vi "HFRR ADV v013 new software.vi"() -> ()   [LabVIEW 2025] (continued)
              n1464 = local write "FRIC. FORCE :"(w1751) -> ()
            }
            frame 1 {
              n1465 = local write "TEMPERATURE :"(w1752) -> ()
            }
            frame 2 {
              n1466 = local write "HUMIDITY:"(w1753) -> ()
            }
            frame 3 {
              n1467 = local write "AIR TEMPERATURE :"(w1754) -> ()
            }
            frame 4 {
              n1468 = local write "Com Port 1"(w1755) -> ()
            }
            frame 5 {
              n1469 = local write "Com Port 2"(w1756) -> ()
              n1470 = local write "visa due"(w1756) -> ()
            }
            frame 6 {
              n1471 = String To Path(string=w1757) -> (path=w1758:path)
              n1472 = local write "File Path"(w1758) -> ()
              "String" <- w1757
            }
            frame 7 {
              n1473 = local write "DISPLACEMENT :"(w1759) -> ()
            }
            frame 8 {
              n1474 = local write "STROKE GAIN :"(w1760) -> ()
            }
            frame 9 {
            }
            frame 10 {
              n1475 = local write "Language Selection"(w1761) -> ()
            }
            frame 11 {
              n1476 = local write "CH-POWER +"(w1762) -> ()
            }
            frame 12 {
              n1477 = local write "CH-POWER -"(w1763) -> ()
            }
            frame 13 {
              n1478 = local write "CH-HEATER"(w1764) -> ()
            }
            frame 14 {
              n1479 = local write "CH-HUMIDITY WET"(w1765) -> ()
            }
            frame 15 {
              n1480 = local write "CH-HUMIDITY DRY"(w1766) -> ()
            }
            frame 16 {
            }
            frame 17 {
              n1481 = local write "AIR TEMP INTERCEPT:"(w1767) -> ()
            }
            frame 18 {
              n1482 = local write "TEMP INTERCEPT:"(w1768) -> ()
            }
            frame 21 {
              n1483 = local write "S.NO"(w1769) -> ()
            }
            frame 22 {
              n1484 = local write "Com Port 3"(w1770) -> ()
            }
            frame 20 {
              n1485 = local write "Camera Port :"(w1771) -> ()
            }
            frame 19 {
              n1486 = local write "C3 :"(w1772) -> ()
            }
            frame 23, Default {
            }
          }
        }
      }
    }
    n1487 = Select(t=u32 2500 ("milliseconds to wait"), s=w1725, f=u32 500 ("milliseconds to wait")) -> (s? t:f=w1723:u32)
    n1488 = Multiply(x=w1728, y=w1723) -> (x*y=w1730:dbl)
    n1489 = property on="Time slide" class="Slide (strict)"("Visible"=w1719) -> ()  [unwired: 2 in, 2 out]
    n1490 = call "Elapsed Time2"("Time Target (s)"=w1730, "Auto Reset"=TRUE) -> ("Time has Elapsed"=w1720:bool)  [unwired: 10 in, 7 out]
    n1491 = case shown="True" w1720 {
      frame False {
      }
      frame True {
        n1492 = stacked-sequence {
          frame #0 {
            # "DATA PROCESSING"
            # "115 mV/N"
            n1493 = local read "Sample Temperature"() -> (w1775:dbl)
            n1494 = local read "RH Numeric:"() -> (w1782:dbl)
            n1495 = local read "HUMIDITY:"() -> (w1783:dbl)
            n1496 = local read "FRICVALZ"() -> (w1794:dbl)
            n1497 = local read "Friction"() -> (w1778:dbl)
            n1498 = Multiply(x=w1782, y=w1783) -> (x*y=→"Humidity ( %RH )" →"Hum" →"Hum 2":dbl)
            n1499 = call <vilib>:"Mean PtByPt.vi"("x"=w1775, "sample length"=100) -> ("mean"=w1774:dbl)  [unwired: 2 in, 1 out]
            "TEMP 2" <- w1774
            "TEMP 3" <- w1774
            n1500 = Subtract(x=w1778, y=w1794) -> (x-y=w1789:dbl)
            "FF 2" <- w1789
            "FF 4" <- w1789
            n1501 = local read "Ambient Temperature"() -> (→"AIR TEMP":dbl)
            n1502 = local read "TEMP"() -> (w1793:dbl)
            n1503 = local write "FF 3"(w1789) -> ()
            n1504 = Compound Arithmetic op=OR("FRICVALZ 4", "FRICVALZ 3", "FRICVALZ 2") -> (w1785:bool)
            n1505 = case shown="True" w1785 {
              tunnel: w1778 -> [_ w1800]
              frame False {
              }
              frame True {
                w1799 = FALSE ("FRICVALZ")
                n1506 = local write "FRICVALZ 3"(w1799) -> ()
                n1507 = local write "FRICVALZ 2"(w1799) -> ()
                n1508 = local write "FRICVALZ 4"(w1799) -> ()
                "FRICVALZ" <- w1800
              }
            }
            n1509 = Not A Number/Path/Refnum?(number/path/refnum=w1793) -> (NaN/Path/Refnum?=w1792:bool)
            n1510 = Not A Number/Path/Refnum?(number/path/refnum=w1789) -> (NaN/Path/Refnum?=w1791:bool)
            n1511 = Divide(x=w1789, y=1.96) -> (x/y=w1786:dbl)
            n1512 = Compound Arithmetic op=OR(w1792, w1791) -> (w1790:bool)
            n1513 = Not A Number/Path/Refnum?(number/path/refnum=w1786) -> (NaN/Path/Refnum?=w1787:bool)
            n1514 = case shown="True" w1790 {
              frame False {
              }
              frame True {
                n1515 = local write "TEMP"(0.0 ("TEMP")) -> ()
                n1516 = local write "FF 2"(0.0 ("FF 2")) -> ()
                n1517 = local write "reinit"(TRUE ("reinit")) -> ()
              }
            }
            n1518 = local write "TEMP"(w1774) -> ()
            n1519 = Select(t=0.0, s=w1787, f=w1786) -> (s? t:f=w1777:dbl)
            "COF 2" <- w1777
            n1520 = local write "COF 3"(w1777) -> ()
          }
        }
      }
    }
    n1521 = Wait (ms)(milliseconds to wait=u32 50) -> ()  [unwired: 1 out]
    n1522 = local read "Quit"() -> (w1712:bool)
    "Rate" <- 2500.0 ("No of Samples")
  }
  n1523 = while {
    tunnel: w57 -> [_]
    tunnel: [w1827] -> _
    tunnel: [w1803] -> w56
    i -> [w1827]
    stop <- w1803 stop-if-true
    # "C:\\LAB-IQ-NXT\\Scar View.exe"
    n1524 = local read "OK Button 16"() -> (w1816:bool)
    n1525 = local read "Main Tab"() -> (w1809:T2)
    n1526 = local read "service 3"() -> (w1810:bool)
    n1527 = local read "OPEN 6"() -> (w1812:bool)
    n1528 = local read "EDIT 2"() -> (w1814:bool)
    n1529 = flat-sequence {
      frame #0 {
        n1530 = local read "SAVE 2"() -> (w2429:bool)
        n1531 = stacked-sequence {
          frame #0 {
            n1532 = local read "EDIT"() -> (w2483:bool)
            n1533 = case shown="True" w2483 {
              tunnel: [u8 2 ("Disabled") u8 0 ("Disabled")] -> _
              frame False {
                w2485 = FALSE
                n1534 = local write "Password"("") -> ()
                n1535 = property on="SrvM CP" class="Bool (strict)"("Visible"=w2485) -> ()  [unwired: 2 in, 2 out]
                n1536 = property on="message" class="Str"("Visible"=w2485) -> ()  [unwired: 2 in, 2 out]
                n1537 = local write "x = y?"(w2485) -> ()
                n1538 = property on="Password" class="Str"("Visible"=w2485) -> ()  [unwired: 2 in, 2 out]
                n1539 = property on="ENTER THE NEW PASSWORD" class="Str"("Visible"=w2485) -> ()  [unwired: 2 in, 2 out]
                n1540 = property on="ENTER CURRENT PASSWORD" class="Str"("Visible"=w2485) -> ()  [unwired: 2 in, 2 out]
                n1541 = local write "SrvM CP"(w2485) -> ()
              }
              frame True {
                w2488 = TRUE
                n1542 = property on="SrvM CP" class="Bool (strict)"("Visible"=w2488) -> ()  [unwired: 2 in, 2 out]
                n1543 = property on="Password" class="Str"("Visible"=w2488) -> ()  [unwired: 2 in, 2 out]
              }
            }
            "dipl pwd" <- "@143$\n" ("dipl pwd")
          }
          frame #1 {
            # "Gain password"
            n1544 = String To Byte Array(string="ENTER CURRENT PASSWORD") -> (unsigned byte array=w2493:u8[])
            n1545 = Search 1D Array(1D array=w2493, element=u8 10) -> (index of element=w2496:i32)  [unwired: 1 in]
            n1546 = Index Array(array=w2493, index=w2496) -> (element=w2492:u8)
            n1547 = Equal?(x=w2492, y=10) -> (x = y?=w2490:bool)
            n1548 = case shown="True" w2490 {
              frame False {
                n1549 = property on="ENTER THE NEW PASSWORD" class="Str"("Visible"=FALSE) -> ()  [unwired: 2 in, 2 out]
              }
              frame True {
                # "password"
                # "change password logic"
                n1550 = local read "ENTER CURRENT PASSWORD"() -> (w2509:string)
                n1551 = local read "dipl pwd"() -> (w2503:string)
                n1552 = String To Byte Array(string=w2509) -> (unsigned byte array=w2511:u8[])
                n1553 = String To Byte Array(string=w2503) -> (unsigned byte array=w2504:u8[])
                n1554 = Array Size(array=w2511) -> (size(s)=w2508:i32)
                n1555 = Array Size(array=w2504) -> (size(s)=w2506:i32)
                n1556 = for {
                  N: w2508 -> [_]
                  tunnel: w2511 -> [w2535]
                  tunnel: [w2533] -> w2512 mode=indexing
                  tunnel: w2508 -> [w2527]
                  i -> [w2528]
                  n1557 = Decrement(x=w2527) -> (x-1=w2525:i32)
                  n1558 = Equal?(x=w2528, y=w2525) -> (x = y?=w2526:bool)
                  n1559 = Index Array(array=w2535, index=w2528) -> (element=w2529:u8)
                  n1560 = Number To Decimal String(number=w2529) -> (decimal integer string=w2534:string)  [unwired: 1 in]
                  n1561 = Select(t="", s=w2526, f="\r") -> (s? t:f=w2531:string)
                  n1562 = Concatenate Strings(w2534, w2531) -> (w2533:string)
                }
                n1563 = for {
                  N: w2506 -> [_]
                  tunnel: w2504 -> [w2523]
                  tunnel: [w2521] -> w2505 mode=indexing
                  tunnel: w2506 -> [w2518]
                  i -> [w2519]
                  n1564 = Decrement(x=w2518) -> (x-1=w2517:i32)
                  n1565 = Equal?(x=w2519, y=w2517) -> (x = y?=w2516:bool)
                  n1566 = Index Array(array=w2523, index=w2519) -> (element=w2522:u8)
                  n1567 = Number To Decimal String(number=w2522) -> (decimal integer string=w2520:string)  [unwired: 1 in]
                  n1568 = Select(t="", s=w2516, f="\r") -> (s? t:f=w2513:string)
                  n1569 = Concatenate Strings(w2520, w2513) -> (w2521:string)
                }
                n1570 = local read "string"() -> (w2510:string)
                n1571 = Concatenate Strings(w2505) -> (w2499:string)
                n1572 = Concatenate Strings(w2510) -> (w2507:string)
                n1573 = Concatenate Strings(w2512) -> (w2500:string)
                n1574 = Equal?(x=w2500, y=w2507) -> (x = y?=w2502:bool)
                n1575 = Equal?(x=w2500, y=w2499) -> (x = y?=w2498:bool)
                n1576 = Or(x=w2502, y=w2498) -> (x .or. y?=w2501:bool)
                n1577 = case shown="True" w2501 {
                  frame False {
                  }
                  frame True {
                    n1578 = property on="ENTER THE NEW PASSWORD" class="Str"("Visible"=TRUE) -> ()  [unwired: 2 in, 2 out]
                  }
                }
              }
            }
          }
          frame #2 {
            n1579 = String To Byte Array(string="ENTER THE NEW PASSWORD") -> (unsigned byte array=w2538:u8[])
            n1580 = Search 1D Array(1D array=w2538, element=u8 10) -> (index of element=w2542:i32)  [unwired: 1 in]
            n1581 = Index Array(array=w2538, index=w2542) -> (element=w2540:u8)
            n1582 = Equal?(x=w2540, y=10) -> (x = y?=w2537:bool)
            n1583 = case shown="False" w2537 {
              frame False {
              }
              frame True {
                n1584 = local write "EDIT"(FALSE) -> ()
                n1585 = local write "SrvM CP"(FALSE) -> ()
                n1586 = local read "ENTER THE NEW PASSWORD"() -> (w2545:string)
                n1587 = String To Byte Array(string=w2545) -> (unsigned byte array=w2550:u8[])
                n1588 = Array Size(array=w2550) -> (size(s)=w2547:i32)
                n1589 = for {
                  N: w2547 -> [_]
                  tunnel: w2550 -> [w2563]
                  tunnel: [w2560] -> w2552 mode=indexing
                  tunnel: w2547 -> [w2555]
                  i -> [w2553]
                  n1590 = Decrement(x=w2555) -> (x-1=w2556:i32)
                  n1591 = Equal?(x=w2553, y=w2556) -> (x = y?=w2557:bool)
                  n1592 = Index Array(array=w2563, index=w2553) -> (element=w2562:u8)
                  n1593 = Number To Decimal String(number=w2562) -> (decimal integer string=w2561:string)  [unwired: 1 in]
                  n1594 = Select(t="", s=w2557, f="\r") -> (s? t:f=w2554:string)
                  n1595 = Concatenate Strings(w2561, w2554) -> (w2560:string)
                }
                n1596 = local read "file path"() -> (w2544:path)
                n1597 = Concatenate Strings(w2552) -> (w2546:string)
                n1598 = Delete(path (use dialog)=w2544) -> (deleted path=w2548:path)  [unwired: 4 in, 2 out]
                n1599 = call <vilib>:"Write Characters To File.vi"("append to file? (new file:F)"=FALSE, "character string"=w2546, "file path (dialog if empty)"=w2548) -> ()  [unwired: 2 in, 1 out]
              }
            }
          }
          frame #3 {
            n1600 = case shown="True" "SrvM CP" {
              frame False {
                w2566 = ""
                n1601 = local write "ENTER CURRENT PASSWORD"(w2566) -> ()
                n1602 = local write "ENTER THE NEW PASSWORD"(w2566) -> ()
                n1603 = property on="ENTER CURRENT PASSWORD" class="Str"("Visible"=FALSE) -> ()  [unwired: 2 in, 2 out]
              }
              frame True {
                n1604 = property on="ENTER THE NEW PASSWORD" class="Str"() -> ("Visible"=w2567:bool)  [unwired: 2 in, 2 out]
                n1605 = Not(x=w2567) -> (.not. x?=w2568:bool)
                n1606 = property on="ENTER CURRENT PASSWORD" class="Str"("Visible"=w2568) -> ()  [unwired: 2 in, 2 out]
              }
            }
          }
          frame #4 {
            n1607 = String To Byte Array(string="Password") -> (unsigned byte array=w2575:u8[])
            n1608 = Search 1D Array(1D array=w2575, element=u8 10) -> (index of element=w2573:i32)  [unwired: 1 in]
            n1609 = Index Array(array=w2575, index=w2573) -> (element=w2574:u8)
            n1610 = Equal?(x=w2574, y=10) -> (x = y?=w2570:bool)
            n1611 = case shown="True" w2570 {
              frame False {
              }
              frame True {
                # "password"
                # "password"
                n1612 = local read "Password"() -> (w2588:string)
                n1613 = String To Byte Array(string=w2588) -> (unsigned byte array=w2591:u8[])
                n1614 = String To Byte Array(string="@143$\n") -> (unsigned byte array=w2577:u8[])
                n1615 = Array Size(array=w2591) -> (size(s)=w2586:i32)
                n1616 = Array Size(array=w2577) -> (size(s)=w2582:i32)
                n1617 = for {
                  N: w2586 -> [_]
                  tunnel: w2591 -> [w2625]
                  tunnel: [w2623] -> w2592 mode=indexing
                  tunnel: w2586 -> [w2620]
                  i -> [w2621]
                  n1618 = Decrement(x=w2620) -> (x-1=w2619:i32)
                  n1619 = Index Array(array=w2625, index=w2621) -> (element=w2624:u8)
                  n1620 = Equal?(x=w2621, y=w2619) -> (x = y?=w2618:bool)
                  n1621 = Number To Decimal String(number=w2624) -> (decimal integer string=w2622:string)  [unwired: 1 in]
                  n1622 = Select(t="", s=w2618, f="\r") -> (s? t:f=w2615:string)
                  n1623 = Concatenate Strings(w2622, w2615) -> (w2623:string)
                }
                n1624 = for {
                  N: w2582 -> [_]
                  tunnel: w2577 -> [w2636]
                  tunnel: [w2634] -> w2580 mode=indexing
                  tunnel: w2582 -> [w2631]
                  i -> [w2632]
                  n1625 = Decrement(x=w2631) -> (x-1=w2630:i32)
                  n1626 = Index Array(array=w2636, index=w2632) -> (element=w2635:u8)
                  n1627 = Equal?(x=w2632, y=w2630) -> (x = y?=w2629:bool)
                  n1628 = Number To Decimal String(number=w2635) -> (decimal integer string=w2633:string)  [unwired: 1 in]
                  n1629 = Select(t="", s=w2629, f="\r") -> (s? t:f=w2626:string)
                  n1630 = Concatenate Strings(w2633, w2626) -> (w2634:string)
                }
                n1631 = local read "file path"() -> (w2576:path)
                n1632 = call <vilib>:"Read Characters From File.vi"("file path (dialog if empty)"=w2576) -> ("character string"=w2590:string)  [unwired: 5 in, 3 out]
                "string" <- w2590
                n1633 = flat-sequence {
                  tunnel: [w2593] -> w2587
                  frame #0 {
                    w2593 = ""
                    n1634 = local write "Password"(w2593) -> ()
                  }
                }
                n1635 = Concatenate Strings(w2580) -> (w2581:string)
                n1636 = Concatenate Strings(w2590) -> (w2589:string)
                n1637 = Concatenate Strings(w2592) -> (w2584:string)
                n1638 = Equal?(x=w2584, y=w2589) -> (x = y?=w2579:bool)
                n1639 = Equal?(x=w2584, y=w2581) -> (x = y?=w2585:bool)
                n1640 = Or(x=w2579, y=w2585) -> (x .or. y?=w2578:bool)
                "x = y?" <- w2578
                n1641 = case shown="True" w2578 {
                  selector: w2578 -> [w2595 _]
                  tunnel: w2587 -> [_ _]
                  frame False {
                    n1642 = And(x=w2595, y=TRUE ("Visible")) -> (x .and. y?=w2596:bool)
                    n1643 = property on="message" class="Str"("Visible"=w2596) -> ()  [unwired: 2 in, 2 out]
                  }
                  frame True {
                    n1644 = control-ref of="This VI"() -> (w2607:refnum<vi>)
                    n1645 = property class="VI"(reference=w2607) -> (reference out=w2598:refnum<vi>, error out=w2602:errorcluster, "Panel"=w2606:refnum<vi>)  [unwired: 1 in]
                    n1646 = property on="message" class="Str"("Visible"=FALSE) -> ()  [unwired: 2 in, 2 out]
                    n1647 = property class="Pnl"(reference=w2606, error in=w2602) -> (reference out=w2600:refnum<vi>, error out=w2603:errorcluster, "Panes[]"=w2605:refnum<vi>[])
                    n1648 = for {
                      tunnel: w2605 -> [w2614] mode=indexing
                      tunnel: T20."Always On" ("Horizontal Scrollbar Visibility") -> [w2613]
                      tunnel: w2603 -> [w2610]
                      tunnel: [w2609] -> w2601
                      n1649 = property class="Pane"(reference=w2614, error in=w2610, "HorizScrollbarVisibility"=w2613) -> (reference out=w2611:refnum<vi>, error out=w2612:errorcluster)
                      n1650 = Close Reference(reference=w2611, error in (no error)=w2612) -> (error out=w2609:errorcluster)
                    }
                    n1651 = Close Reference(reference=w2600, error in (no error)=w2601) -> (error out=w2599:errorcluster)
                    n1652 = Close Reference(reference=w2598, error in (no error)=w2599) -> (error out=→"error out 6":errorcluster)
                  }
                }
              }
            }
          }
        }
        n1653 = local read "x = y?"() -> (w2435:bool)
        n1654 = local read "HUMIDITY: 2"() -> (w2437:dbl)
        n1655 = local read "HUMIDITY:"() -> (w2436:dbl)
        n1656 = property on="Port 2 Error" class="Clust (strict)"("Visible"="EDIT") -> ()  [unwired: 2 in, 2 out]
        n1657 = property on="Port 1 Error" class="Clust (strict)"("Visible"="EDIT") -> ()  [unwired: 2 in, 2 out]
        n1658 = case shown="True" "SrvM CP 2" {
          frame False {
          }
          frame True {
            n1659 = local write "SrvM CP 2"(FALSE ("SrvM CP 2")) -> ()
            n1660 = local read "HUMIDITY: 2"() -> (w2476:dbl)
            n1661 = local read "TEMP INTERCEPT: 2"() -> (w2475:dbl)
            n1662 = local read "DISPLACEMENT : 4"() -> (w2479:dbl)
            n1663 = local read "TEMPERATURE : 2"() -> (w2478:dbl)
            n1664 = local read "STROKE GAIN : 2"() -> (w2480:dbl)
            n1665 = local read "FRIC. FORCE : 2"() -> (w2481:dbl)
            n1666 = local read "AIR TEMP INTERCEPT: 2"() -> (w2474:dbl)
            n1667 = local read "AIR TEMPERATURE : 2"() -> (w2477:dbl)
            n1668 = local write "HUMIDITY:"(w2476) -> ()
            n1669 = local write "AIR TEMP INTERCEPT:"(w2475) -> ()
            n1670 = local write "TEMPERATURE :"(w2478) -> ()
            n1671 = local write "FRIC. FORCE :"(w2481) -> ()
            n1672 = local write "STROKE GAIN :"(w2480) -> ()
            n1673 = local write "DISPLACEMENT :"(w2479) -> ()
            n1674 = local write "AIR TEMPERATURE :"(w2477) -> ()
            n1675 = local write "TEMP INTERCEPT:"(w2474) -> ()
          }
        }
        n1676 = Or(x="SAVE", y=w2429) -> (x .or. y?=w2430:bool)
        n1677 = And(x="EDIT", y=w2435) -> (x .and. y?=w2433:bool)
        n1678 = local read "DISPLACEMENT : 4"() -> (w2446:dbl)
        n1679 = local read "TEMPERATURE : 2"() -> (w2444:dbl)
        n1680 = local read "STROKE GAIN : 2"() -> (w2450:dbl)
        n1681 = local read "DISPLACEMENT :"() -> (w2445:dbl)
        n1682 = local read "FRIC. FORCE : 2"() -> (w2453:dbl)
        n1683 = local read "TEMPERATURE :"() -> (w2442:dbl)
        n1684 = local read "STROKE GAIN :"() -> (w2449:dbl)
        n1685 = local read "FRIC. FORCE :"() -> (w2452:dbl)
        n1686 = case shown="True" w2433 {
          tunnel: [u8 2 ("Disabled") u8 0 ("Disabled")] -> w2432
          tunnel: [w2797 TRUE ("Visible")] -> w2431
          frame False {
            w2797 = FALSE ("Visible")
            n1687 = local write "EDIT 2"(w2797) -> ()
          }
          frame True {
          }
        }
        n1688 = case shown="True" w2430 {
          frame False {
          }
          frame True {
            n1689 = stacked-sequence {
              seq-local: [w2645 _ _] -> [_ w2792 _]
              frame #0 {
                (unwired) i16 5 ("precision (6)")
                # "[CH1]    - FF\n[CH2]   - TEMPERATURE\n[CH3]    - Humidity\n[CH4]    - AIR TEMP\n[CH5]\\- Visa Uno\n[CH6] \\- Visa Due\n[CH7]  \\- file path\n[CH8]   - Displacement Gain\n[CHA]   - Stroke Gain\n[CHB]   - Stroke PID Gain\n[CHC]   -Language Selection\n[CHD]   -Power +\n[CHE]   -Power_\n[CHF]   -Heater\n[CHG]   -Humidity Wet\n[CHH]   -Humidity Dry\n[CHI]   -Integral Time"
                n1690 = local read "Language Selection"() -> (w2693:enum16{"English", "Russian"})
                n1691 = local read "CH-HUMIDITY WET"() -> (w2651:u16)
                n1692 = local read "CH-HUMIDITY DRY"() -> (w2648:u16)
                n1693 = local read "STROKE GAIN :"() -> (w2637:dbl)
                n1694 = local read "CH-POWER +"() -> (w2660:u16)
                n1695 = local read "CH-POWER -"() -> (w2657:u16)
                n1696 = local read "CH-HEATER"() -> (w2654:u16)
                n1697 = local read "AIR TEMPERATURE :"() -> (w2640:dbl)
                n1698 = local read "DISPLACEMENT :"() -> (w2638:dbl)
                n1699 = local read "TEMPERATURE :"() -> (w2641:dbl)
                n1700 = local read "FRIC. FORCE :"() -> (w2642:dbl)
                n1701 = local read "HUMIDITY:"() -> (w2639:dbl)
                n1702 = Path To String(path="File Path") -> (string=w2709:string)
                n1703 = Number To Fractional String(number=w2637, width (-)=i16 10 ("precision (6)"), precision (6)=i16 5) -> (F-format string=w2700:string)  [unwired: 1 in]
                n1704 = Number To Fractional String(number=w2693, width (-)=i16 10 ("precision (6)"), precision (6)=i16 5) -> (F-format string=w2689:string)  [unwired: 1 in]
                n1705 = Number To Fractional String(number=w2660, width (-)=i16 10 ("precision (6)"), precision (6)=i16 5) -> (F-format string=w2683:string)  [unwired: 1 in]
                n1706 = Number To Fractional String(number=w2657, width (-)=i16 10 ("precision (6)"), precision (6)=i16 5) -> (F-format string=w2680:string)  [unwired: 1 in]
                n1707 = Number To Fractional String(number=w2654, width (-)=i16 10 ("precision (6)"), precision (6)=i16 5) -> (F-format string=w2675:string)  [unwired: 1 in]
                n1708 = Number To Fractional String(number=w2651, width (-)=i16 10 ("precision (6)"), precision (6)=i16 5) -> (F-format string=w2672:string)  [unwired: 1 in]
                n1709 = Number To Fractional String(number=w2648, width (-)=i16 10 ("precision (6)"), precision (6)=i16 5) -> (F-format string=w2667:string)  [unwired: 1 in]
                n1710 = local read "Com Port 1"() -> (w2644:refnum<visa-resource-name>)
                n1711 = local read "Com Port 2"() -> (w2643:refnum<visa-resource-name>)
                n1712 = Concatenate Strings(w2709, "\\" ("string")) -> (w2708:string)
                n1713 = Number To Fractional String(number=w2642, width (-)=i16 10 ("precision (6)"), precision (6)=i16 5) -> (F-format string=w2741:string)  [unwired: 1 in]
                n1714 = Number To Fractional String(number=w2641, width (-)=i16 10 ("precision (6)"), precision (6)=i16 5) -> (F-format string=w2740:string)  [unwired: 1 in]
                n1715 = Number To Fractional String(number=w2639, width (-)=i16 10 ("precision (6)"), precision (6)=i16 5) -> (F-format string=w2734:string)  [unwired: 1 in]
                n1716 = Number To Fractional String(number=w2640, width (-)=i16 10 ("precision (6)"), precision (6)=i16 5) -> (F-format string=w2728:string)  [unwired: 1 in]
                n1717 = Number To Fractional String(number=w2638, width (-)=i16 10 ("precision (6)"), precision (6)=i16 5) -> (F-format string=w2701:string)  [unwired: 1 in]
                n1718 = Concatenate Strings("[CHA]" ("string"), w2700, "- Stroke Gain" ("string"), "\r") -> (w2694:string)
                n1719 = Concatenate Strings("[CHC]" ("string"), w2689, "-Language Selection" ("string"), "\r") -> (w2686:string)
                n1720 = Concatenate Strings("[CHD]" ("string"), w2683, "-Power +" ("string"), "\r") -> (w2665:string)
                n1721 = Concatenate Strings("[CHG]" ("string"), w2672, "-Humidity Wet" ("string"), "\r") -> (w2662:string)
                n1722 = Concatenate Strings("[CHH]" ("string"), w2667, "-Humidity Dry" ("string"), "\r") -> (w2661:string)
                n1723 = Concatenate Strings("[CH1]" ("string"), w2741, " - FF" ("string"), "\r") -> (w2739:string)
                n1724 = Concatenate Strings("[CH2]" ("string"), w2740, " - TEMPERATURE" ("string"), "\r") -> (w2738:string)
                n1725 = Concatenate Strings("[CH3]" ("string"), w2734, " - Humidity" ("string"), "\r") -> (w2731:string)
                n1726 = Concatenate Strings("[CH4]" ("string"), w2728, " - AIR TEMP" ("string"), "\r") -> (w2724:string)
                n1727 = Concatenate Strings("[CH5]" ("string"), w2644, "- Visa Uno" ("string"), "\r") -> (w2717:string)
                n1728 = Concatenate Strings("[CH6]" ("string"), w2643, "- Visa Due" ("string"), "\r") -> (w2712:string)
                n1729 = Concatenate Strings("[CH7]" ("string"), w2708, "- file path" ("string"), "\r") -> (w2711:string)
                n1730 = Concatenate Strings("[CH8]" ("string"), w2701, "- Displacement Gain" ("string"), "\r") -> (w2704:string)
                n1731 = Concatenate Strings("[CHE]" ("string"), w2680, "-Power_" ("string"), "\r") -> (w2664:string)
                n1732 = Concatenate Strings("[CHF]" ("string"), w2675, "-Heater" ("string"), "\r") -> (w2663:string)
                n1733 = Concatenate Strings(w2739, w2738, w2731, w2724, w2717, w2712, w2711, w2704, w2694, w2686, w2665, w2664, w2663, w2662, w2661) -> (w2645:string)
                "gain" <- w2645
              }
              frame #1 {
                n1734 = local read "Camera Port :"() -> (w2753:string)
                n1735 = local read "C3 :"() -> (w2761:refnum<visa-resource-name>)
                n1736 = local read "TEMP INTERCEPT:"() -> (w2762:dbl)
                n1737 = local read "AIR TEMP INTERCEPT:"() -> (w2763:dbl)
                n1738 = local read "Com Port 3"() -> (w2764:refnum<visa-resource-name>)
                n1739 = Concatenate Strings("[CH8]" ("string"), w2753, "- Visa Camera" ("string"), "\r") -> (w2752:string)
                n1740 = Concatenate Strings("[CH7]" ("string"), w2761, "- Visa Humidity" ("string"), "\r") -> (w2757:string)
                n1741 = Number To Fractional String(number=w2762, width (-)=i16 10 ("precision (6)"), precision (6)=i16 5) -> (F-format string=w2780:string)  [unwired: 1 in]
                n1742 = Concatenate Strings("[CHL]" ("string"), w2764, "- Visa humid" ("string"), "\r") -> (w2767:string)
                n1743 = Number To Fractional String(number=w2763, width (-)=i16 10 ("precision (6)"), precision (6)=i16 5) -> (F-format string=w2787:string)  [unwired: 1 in]
                n1744 = Concatenate Strings("[CHK]" ("string"), w2780, "-TEMP INTERCEPT" ("string"), "\r") -> (w2776:string)
                n1745 = Concatenate Strings("[SNO]" ("string"), "S.NO", "-" ("string"), "\r") -> (w2772:string)
                n1746 = Concatenate Strings("[CHJ]" ("string"), w2787, "-AIR TEMP INTERCEPT" ("string"), "\r") -> (w2777:string)
                n1747 = String To Path(string="C:\\LAB-IQ\\calibrate WO 2465.dcf") -> (path=w2765:path)
                n1748 = Concatenate Strings(w2792, w2777, w2776, w2772, w2767, w2757, w2752) -> (w2791:string)
                n1749 = call <vilib>:"Write Characters To File.vi"("append to file? (new file:F)"=FALSE, "character string"=w2791, "file path (dialog if empty)"=w2765) -> ()  [unwired: 2 in, 1 out]
              }
              frame #2 {
                n1750 = local write "Lan flag"(0.0 ("Lan flag")) -> ()
                n1751 = local write "conststatus"(0.0 ("rpm value : 2")) -> ()
                n1752 = local write "SAVE"(FALSE ("OK Button 14")) -> ()
                n1753 = local write "SAVE 2"(FALSE ("SAVE 2")) -> ()
              }
            }
          }
        }
        n1754 = Subtract(x=w2437, y=w2436) -> (x-y=w2438:dbl)
        n1755 = local read "AIR TEMPERATURE : 2"() -> (w2441:dbl)
        n1756 = local read "AIR TEMPERATURE :"() -> (w2440:dbl)
        n1757 = Divide(x=w2438, y=w2436) -> (x/y=w2460:dbl)
        n1758 = Subtract(x=w2453, y=w2452) -> (x-y=w2451:dbl)
        n1759 = Subtract(x=w2444, y=w2442) -> (x-y=w2443:dbl)
        n1760 = Subtract(x=w2450, y=w2449) -> (x-y=w2448:dbl)
        n1761 = Subtract(x=w2446, y=w2445) -> (x-y=w2447:dbl)
        n1762 = Subtract(x=w2441, y=w2440) -> (x-y=w2439:dbl)
        n1763 = Divide(x=w2451, y=w2452) -> (x/y=w2471:dbl)
        n1764 = Divide(x=w2443, y=w2442) -> (x/y=w2464:dbl)
        n1765 = Divide(x=w2448, y=w2449) -> (x/y=w2468:dbl)
        n1766 = Divide(x=w2447, y=w2445) -> (x/y=w2467:dbl)
        n1767 = Multiply(x=w2460, y=100.0) -> (x*y=→"HUMIDITY  Calibration Error":dbl)
        n1768 = Divide(x=w2439, y=w2440) -> (x/y=w2463:dbl)
        n1769 = Multiply(x=w2471, y=100.0) -> (x*y=→"FRIC. FORCE Calibration Error":dbl)
        n1770 = Multiply(x=w2464, y=100.0) -> (x*y=→"TEMPERATURE  Calibration Error":dbl)
        n1771 = Multiply(x=w2468, y=100.0) -> (x*y=→"STROKE Calibration Error":dbl)
        n1772 = Multiply(x=w2467, y=100.0) -> (x*y=→"DISPLACEMENT  Calibration Error":dbl)
        n1773 = property on="EDIT 2" class="Bool (strict)"("Visible"=w2431) -> ()  [unwired: 2 in, 2 out]
        n1774 = property on="SAVE" class="Bool (strict)"("Visible"=w2431) -> ()  [unwired: 2 in, 2 out]
        n1775 = property on="SrvM CP" class="Bool (strict)"("Disabled"=w2432) -> ()  [unwired: 2 in, 2 out]
        n1776 = property on="visa due" class="CmbBox"("Disabled"=w2432) -> ()  [unwired: 2 in, 2 out]
        n1777 = property on="File Path" class="Path"("Disabled"=w2432) -> ()  [unwired: 2 in, 2 out]
        n1778 = Multiply(x=w2463, y=100.0) -> (x*y=→"AIR TEMPERATURE  Calibration Error":dbl)
        n1779 = property on="Language Selection" class="Enum (strict)"("Visible"=w2431) -> ()  [unwired: 2 in, 2 out]
        n1780 = property on="Tab Control 7" class="TabCtl (strict)"("Disabled"=w2432) -> ()  [unwired: 2 in, 2 out]
        n1781 = property on="AIR TEMP INTERCEPT:" class="DigNum (strict)"("Disabled"=w2432) -> ()  [unwired: 2 in, 2 out]
        n1782 = property on="CH-POWER -" class="DigNum (strict)"("Disabled"=w2432) -> ()  [unwired: 2 in, 2 out]
        n1783 = property on="CH-POWER +" class="DigNum (strict)"("Disabled"=w2432) -> ()  [unwired: 2 in, 2 out]
        n1784 = property on="AIR TEMPERATURE :" class="DigNum (strict)"("Disabled"=w2432) -> ()  [unwired: 2 in, 2 out]
        n1785 = property on="STROKE GAIN :" class="DigNum (strict)"("Disabled"=w2432) -> ()  [unwired: 2 in, 2 out]
        n1786 = property on="SPEED OUT:" class="DigNum (strict)"("Disabled"=w2432) -> ()  [unwired: 2 in, 2 out]
        n1787 = property on="CH-HUMIDITY DRY" class="DigNum (strict)"("Disabled"=w2432) -> ()  [unwired: 2 in, 2 out]
        n1788 = property on="HUMIDITY:" class="DigNum (strict)"("Disabled"=w2432) -> ()  [unwired: 2 in, 2 out]
        n1789 = property on="CH-HUMIDITY WET" class="DigNum (strict)"("Disabled"=w2432) -> ()  [unwired: 2 in, 2 out]
        n1790 = property on="TEMPERATURE :" class="DigNum (strict)"("Disabled"=w2432) -> ()  [unwired: 2 in, 2 out]
        n1791 = property on="DISPLACEMENT :" class="DigNum (strict)"("Disabled"=w2432) -> ()  [unwired: 2 in, 2 out]
        n1792 = property on="CH-HEATER" class="DigNum (strict)"("Disabled"=w2432) -> ()  [unwired: 2 in, 2 out]
        n1793 = property on="TEMP INTERCEPT:" class="DigNum (strict)"("Disabled"=w2432) -> ()  [unwired: 2 in, 2 out]
        n1794 = property on="FRIC. FORCE :" class="DigNum (strict)"("Disabled"=w2432) -> ()  [unwired: 2 in, 2 out]
      }
    }
    n1795 = local read "RUN"() -> (w1826:bool)
    n1796 = local read "RUN"() -> (w1824:bool)
    n1797 = disable-structure shown="Disabled" {
      disable-tunnel: [w1841 _] -> w1807
      disable-tunnel: [w1840 _] -> w1805
      frame Disabled {
        n1798 = local read "Temperature before test"() -> (w1834:dbl)
        n1799 = local read "Temperature after test"() -> (w1847:dbl)
        n1800 = case shown="True" "Save Results" {
          frame False {
          }
          frame True {
            w1863 = "\r"
            n1801 = local write "Save Results"(FALSE ("OK Button 5")) -> ()
            n1802 = local read "Temperature before test"() -> (w1901:dbl)
            n1803 = local read "Temperature after test"() -> (w1903:dbl)
            n1804 = local read "Humidity before test"() -> (w1900:dbl)
            n1805 = local read "Humidity after test"() -> (w1902:dbl)
            n1806 = local read "WS1.4"() -> (w1907:dbl)
            n1807 = local read "AVP"() -> (w1905:dbl)
            n1808 = Number To Fractional String(number=w1907, width (-)=i16 6, precision (6)=i16 1) -> (F-format string=w1867:string)  [unwired: 1 in]
            n1809 = local read "MWSD"() -> (w1904:dbl)
            n1810 = local read "String"() -> (w1896:string)
            n1811 = local read "FILE"() -> (w1899:string)
            n1812 = local read "HCF"() -> (w1906:dbl)
            n1813 = Number To Fractional String(number=w1900, width (-)=i16 6, precision (6)=i16 1) -> (F-format string=w1892:string)  [unwired: 1 in]
            n1814 = Number To Fractional String(number=w1901, width (-)=i16 6, precision (6)=i16 1) -> (F-format string=w1889:string)  [unwired: 1 in]
            n1815 = Number To Fractional String(number=w1902, width (-)=i16 6, precision (6)=i16 1) -> (F-format string=w1885:string)  [unwired: 1 in]
            n1816 = Number To Fractional String(number=w1903, width (-)=i16 6, precision (6)=i16 1) -> (F-format string=w1881:string)  [unwired: 1 in]
            n1817 = Number To Fractional String(number=w1905, width (-)=i16 6, precision (6)=i16 3) -> (F-format string=w1874:string)  [unwired: 1 in]
            n1818 = Concatenate Strings(w1896, w1899) -> (w1918:string)
            n1819 = Number To Fractional String(number=w1904, width (-)=i16 6, precision (6)=i16 1) -> (F-format string=w1878:string)  [unwired: 1 in]
            n1820 = Number To Fractional String(number=w1906, width (-)=i16 6, precision (6)=i16 2) -> (F-format string=w1872:string)  [unwired: 1 in]
            n1821 = Concatenate Strings("(" ("string"), w1867, ")Microns" ("string")) -> (w1866:string)
            n1822 = local read "REMARKS"() -> (w1898:string)
            "REMARKS 2" <- w1898
            n1823 = Concatenate Strings("(" ("string"), w1892, " ) % RH," ("string")) -> (w1893:string)
            n1824 = Concatenate Strings(w1872, ")" ("string")) -> (w1870:string)
            n1825 = Concatenate Strings("(" ("string"), w1889, ")  Deg C ," ("string")) -> (w1888:string)
            n1826 = Concatenate Strings("(" ("string"), w1885, " ) % RH," ("string")) -> (w1884:string)
            n1827 = Concatenate Strings("(" ("string"), w1881, ")  Deg C ," ("string")) -> (w1880:string)
            n1828 = Concatenate Strings("(" ("string"), w1878, ")  Microns," ("string")) -> (w1877:string)
            n1829 = Concatenate Strings("(" ("string"), w1874, ")  kPa," ("string")) -> (w1864:string)
            n1830 = Concatenate Strings(w1918, ".dwm" ("Substring")) -> (w1916:string)
            n1831 = String To Path(string=w1916) -> (path=w1915:path)
            n1832 = Concatenate Strings(w1898, w1863, " Humidity before test= " ("Substring"), w1893, w1863, " Temperature before test = " ("Substring"), w1888, w1863, " Humidity after test= " ("Substring"), w1884, w1863, "Temperature after test = " ("Substring"), w1880, w1863, "MSD = " ("Substring"), w1877, w1863, "  AVP = " ("Substring"), w1864, w1863, "  HCF                     =( " ("Substring"), w1870, w1863, " WS1.4                  = " ("Substring"), w1866, w1863) -> (w1862:string)
            "data" <- w1862
            n1833 = call <vilib>:"Write Characters To File.vi"("append to file? (new file:F)"=FALSE, "character string"=w1862, "file path (dialog if empty)"=w1915) -> ()  [unwired: 2 in, 1 out]
            n1834 = Match Pattern(string=w1862, regular expression="!") -> (after substring=→"export":string)  [unwired: 1 in, 3 out]
          }
        }
        n1835 = Add(x=231.864, y=w1834) -> (x+y=w1831:dbl)
        n1836 = Add(x=231.864, y=w1847) -> (x+y=w1844:dbl)
        n1837 = Divide(x=1705.984, y=w1831) -> (x/y=w1832:dbl)
        n1838 = Divide(x=1705.984, y=w1844) -> (x/y=w1845:dbl)
        n1839 = local read "Humidity before test"() -> (w1836:dbl)
        n1840 = local read "Humidity after test"() -> (w1849:dbl)
        n1841 = Subtract(x=8.017352 ("y"), y=w1832) -> (x-y=w1858:dbl)
        n1842 = Subtract(x=8.017352 ("y"), y=w1845) -> (x-y=w1852:dbl)
        n1843 = expression code="10**y"(w1858) -> (w1838:dbl)
        n1844 = expression code="10**y"(w1852) -> (w1851:dbl)
        n1845 = Multiply(x=w1836, y=w1838) -> (x*y=w1837:dbl)
        n1846 = Multiply(x=w1849, y=w1851) -> (x*y=w1850:dbl)
        n1847 = Divide(x=w1837, y=750.0) -> (x/y=w1853:dbl)
        n1848 = Divide(x=w1850, y=750.0) -> (x/y=w1854:dbl)
        n1849 = Add(x=w1853, y=w1854) -> (x+y=w1855:dbl)
        n1850 = Divide(x=w1855, y=2.0) -> (x/y=w1857:dbl)
        n1851 = local write "AVP"(w1857) -> ()
        n1852 = Subtract(x=1.4, y=w1857) -> (x-y=w1840:dbl)
        n1853 = local read "HCF"() -> (w1841:dbl)
      }
      frame Enabled {
      }
    }
    n1854 = case shown="True" "EDIT 3" {
      frame False {
      }
      frame True {
        n1855 = local write "EDIT 3"(FALSE ("EDIT 3")) -> ()
        n1856 = local write "Main Tab"(T2."About" ("Main Tab")) -> ()
      }
    }
    n1857 = case shown="False" w1826 {
      frame False {
        n1858 = local read "stopT"() -> (w2804:bool)
        n1859 = case shown="True" w2804 {
          frame False {
          }
          frame True {
            n1860 = local write "stopT"(FALSE) -> ()
          }
        }
      }
      frame True {
        "stopT" <- TRUE
      }
    }
    n1861 = case shown="False" w1824 {
      frame False {
      }
      frame True {
      }
    }
    n1862 = case shown="True" w1814 {
      frame False {
        n1863 = property on="Password 2" class="Str"("Visible"=FALSE) -> ()  [unwired: 2 in, 2 out]
        n1864 = local write "Password 2"("" ("Password")) -> ()
      }
      frame True {
        n1865 = property on="Password 2" class="Str"("Visible"=TRUE) -> ()  [unwired: 2 in, 2 out]
        n1866 = Equal?(x="Password 2", y="HFRR1234") -> (x = y?=w1946:bool)
        n1867 = case shown="True" w1946 {
          tunnel: "Password 2" -> [w1949 _]
          frame False {
            n1868 = String Length(string=w1949) -> (length=w1950:i32)
            n1869 = Greater Than 0?(x=w1950) -> (x > 0?=w1948:bool)
            n1870 = case shown="False" w1948 {
              frame False {
                n1871 = property on="Password 2" class="Str"("Caption.Text"="Password (Advance Setting)") -> ()  [unwired: 2 in, 2 out]
              }
              frame True {
                n1872 = property on="Password 2" class="Str"("Caption.Text"="Incorrect Password!") -> ()  [unwired: 2 in, 2 out]
              }
            }
          }
          frame True {
            n1873 = local write "EDIT 2"(FALSE ("EDIT 2")) -> ()
            n1874 = local write "Password 2"("" ("Password")) -> ()
            n1875 = local write "Main Tab"(T2."Advance" ("Main Tab")) -> ()
            n1876 = local write "Main Dashboard Buttons"(T1."Advance" ("Main Dashboard Buttons")) -> ()
          }
        }
      }
    }
    n1877 = case shown="True" "Prog Uno" {
      frame False {
      }
      frame True {
        n1878 = stacked-sequence {
          frame #0 {
            n1879 = Delete(path (use dialog)=path "C:/LAB-IQ-NXT/UNOCOMPILE.bat" ("working directory")) -> ()  [unwired: 4 in, 3 out]
          }
          frame #1 {
            n1880 = local read "Com Port 1"() -> (w2411:refnum<visa-resource-name>)
            n1881 = Concatenate Strings("cmd.exe /c \"mode " ("command line"), w2411, ":1200,n,8,1\"\n" ("command line")) -> (w2416:string)
            n1882 = Concatenate Strings(w2416, "CD\\\nCD WinDucom\navrdude -C avrdude.conf -v -patmega328p -carduino -P" ("command line"), w2411, " -b115200 -D -Uflash:w:UNO_V20.hex:i\n" ("command line"), "\r") -> (w2418:string)
            "STR" <- w2418
            n1883 = call <vilib>:"Write Characters To File.vi"("append to file? (new file:F)"=FALSE, "character string"=w2418, "file path (dialog if empty)"=path "C:/LAB-IQ/UNOCOMPILE.bat" ("working directory")) -> ()  [unwired: 2 in, 1 out]
          }
          frame #2 {
            n1884 = disable-structure shown="Disabled" {
              frame Disabled {
                w2422 = "cmd.exe  /c \"C:\\LAB-IQ-NXT\\UNOCOMPILE.bat\"" ("string")
                n1885 = local write "Prog Uno"(FALSE ("run minimized? (F)")) -> ()
                n1886 = call <vilib>:"System Exec.vi"("expected output size  (4096)"=u32 65535, "run minimized? (F)"=FALSE, "wait until completion? (T)"=TRUE ("run minimized? (F)"), "working directory"=path "C:/LAB-IQ-NXT", "standard input"=w2422, "command line"=w2422) -> ("error out"=w2421:errorcluster, "standard output"=→"String 42":string)  [unwired: 2 in, 2 out]
                "error out 3" <- w2421
                n1887 = flat-sequence {
                  tunnel: w2421 -> [_]
                  frame #0 {
                  }
                }
              }
              frame Enabled {
              }
            }
          }
        }
      }
    }
    n1888 = case shown="\"ISO 12156\"" "TEST STANDARD" {
      tunnel: [2.0 ("Set Temp") 0.0 ("Set Temp") 2.0 ("Set Temp") 0.0 ("Set Temp")] -> w1815
      frame "ASTM D6079", Default {
        w2368 = 50.0 ("Hz")
        w2369 = 53.0 ("Set Rh")
        w2371 = 1.0 ("Set Strk")
        w2370 = 60.0 ("Set Temp")
        # "astm hide"
        n1889 = local write "NORMAL LOAD"(200.0 ("NORMAL LOAD")) -> ()
        n1890 = local write "Set Strk"(w2371) -> ()
        n1891 = local write "Set Hz"(w2368) -> ()
        n1892 = local write "Set Temp"(w2370) -> ()
        n1893 = local write "Set Rh"(w2369) -> ()
        n1894 = local write "test time"(75.0 ("test time")) -> ()
        n1895 = local write "Set Stroke:"(w2371) -> ()
        n1896 = local write "Set Humidity:"(w2369) -> ()
        n1897 = local write "Set Frequency:"(w2368) -> ()
        n1898 = local write "Set Temperature:"(w2370) -> ()
        "Test Standard" <- "ASTM D6079" ("Test Standard 2")
      }
      frame "ISO 12156" {
        n1899 = local write "Set Strk"(1.0 ("Set Strk")) -> ()
        n1900 = local write "NORMAL LOAD"(200.0 ("NORMAL LOAD")) -> ()
        n1901 = local write "Set Temp"(60.0 ("Set Temp")) -> ()
        n1902 = local write "test time"(75.0 ("test time")) -> ()
        n1903 = local write "Set Hz"(50.0 ("Hz")) -> ()
        n1904 = local write "Set Rh"(53.0 ("Set Rh")) -> ()
      }
      frame "CEC F-096-A-06" {
        n1905 = local write "Set Strk"(1.0 ("Set Strk")) -> ()
        n1906 = local write "NORMAL LOAD"(200.0 ("NORMAL LOAD")) -> ()
        n1907 = local write "Set Temp"(60.0 ("Set Temp")) -> ()
        n1908 = local write "test time"(75.0 ("test time")) -> ()
        n1909 = local write "Set Hz"(50.0 ("Hz")) -> ()
        n1910 = local write "Set Rh"(53.0 ("Set Rh")) -> ()
      }
      frame "Custom" {
      }
    }
    n1911 = case shown="True" "Prog Due" {
      frame False {
      }
      frame True {
        n1912 = stacked-sequence {
          frame #0 {
            n1913 = Delete(path (use dialog)=path "C:/LAB-IQ/DUECOMPILE.bat" ("working directory")) -> ()  [unwired: 4 in, 3 out]
          }
          frame #1 {
            n1914 = disable-structure shown="Disabled" {
              frame Disabled {
                n1915 = local read "visa due"() -> (w2393:string)
                n1916 = Concatenate Strings("cmd.exe /c \"mode " ("command line"), w2393, ":1200,n,8,1\"\n" ("command line")) -> (w2398:string)
                n1917 = Concatenate Strings(w2398, "CD\\\nCD WinDucom\nTIMEOUT 1\n bossac.exe -i -d --port=" ("command line"), w2393, " -U false -e -w -v -b DUE.bin -R\n" ("command line"), "\r") -> (w2400:string)
                "concatenated string 2" <- w2400
                n1918 = call <vilib>:"Write Characters To File.vi"("append to file? (new file:F)"=FALSE, "character string"=w2400, "file path (dialog if empty)"=path "C:/LAB-IQ-NXT/DUECOMPILE.bat" ("working directory")) -> ()  [unwired: 2 in, 1 out]
              }
              frame Enabled {
              }
            }
          }
          frame #2 {
            # "C:\\LAB-IQ-NXT\\DUECOMPILE.bat"
            n1919 = disable-structure shown="Disabled" {
              frame Disabled {
                w2405 = "cmd.exe  /c \"C:\\LAB-IQ-NXT\\DUECOMPILE.bat\"" ("string")
                n1920 = call <vilib>:"System Exec.vi"("expected output size  (4096)"=u32 65535, "run minimized? (F)"=FALSE, "wait until completion? (T)"=TRUE ("run minimized? (F)"), "working directory"=path "C:/LAB-IQ-NXT", "standard input"=w2405, "command line"=w2405) -> ("error out"=w2404:errorcluster, "standard output"=→"String 44":string)  [unwired: 2 in, 2 out]
                "error out 4" <- w2404
                n1921 = flat-sequence {
                  tunnel: w2404 -> [_]
                  frame #0 {
                  }
                }
              }
              frame Enabled {
              }
            }
            n1922 = local write "Prog Due"(FALSE ("Prog Due")) -> ()
          }
        }
      }
    }
    n1923 = Or(x=w1812, y=w1810) -> (x .or. y?=w1811:bool)
    n1924 = case shown="\"About\"" w1809 {
      tunnel: [T26."Acquire" ("Main Tab") T26."Compare Files" ("Main Tab") T26."About" ("Main Tab")] -> w1822
      frame "Acquire", Default {
      }
      frame "Compare Files" {
      }
      frame "About" {
      }
    }
    n1925 = Or(x=w1816, y="OPEN") -> (x .or. y?=w1817:bool)
    n1926 = case shown="True" w1817 {
      tunnel: w1816 -> [_ w1957]
      frame False {
      }
      frame True {
        n1927 = stacked-sequence {
          tunnel: w1957 -> [_ w2024 _ _]
          frame #0 {
            w1973 = "  " ("String 6")
            n1928 = local write "OPEN"(FALSE ("open")) -> ()
            n1929 = local read "string1 2"() -> (w1961:string)
            n1930 = local read "string1 3"() -> (w1960:string)
            n1931 = local read "string1 4"() -> (w1959:string)
            n1932 = property on="OPEN" class="Bool (strict)"("Visible"=FALSE) -> ()  [unwired: 2 in, 2 out]
            n1933 = local write "String 6"(w1973) -> ()
            n1934 = local write "String 7"(w1973) -> ()
            n1935 = local write "String 8"(w1973) -> ()
            n1936 = local write "String 12"(w1973) -> ()
            n1937 = local read "OK Button 16"() -> (w1958:bool)
            n1938 = String To Path(string=w1961) -> (path=w1969:path)
            n1939 = String To Path(string=w1960) -> (path=w1968:path)
            n1940 = String To Path(string=w1959) -> (path=w1967:path)
            n1941 = case shown="True" w1958 {
              tunnel: [w1974 w1975] -> w1962
              frame False {
                n1942 = local read "string1"() -> (w1974:string)
              }
              frame True {
                n1943 = local read "String Indicator 4"() -> (w1975:string)
              }
            }
            n1944 = Open/Create/Replace File "Open File"(file path (use dialog)=w1969) -> (refnum out=w1965:refnum<file>)  [unwired: 5 in, 2 out]
            n1945 = Open/Create/Replace File "Open File"(file path (use dialog)=w1968) -> (refnum out=w1964:refnum<file>)  [unwired: 5 in, 2 out]
            n1946 = Open/Create/Replace File "Open File"(file path (use dialog)=w1967) -> (refnum out=w1963:refnum<file>)  [unwired: 5 in, 2 out]
            n1947 = while {
              tunnel: w1965 -> [w1987]
              i -> [w1983]
              stop <- w1982 continue-if-true
              (unwired) TRUE ("line mode (F)")
              n1948 = Read from Text File "Read File"(file (use dialog)=w1987) -> (text=w1984:string)  [unwired: 3 in, 3 out]
              n1949 = local write "Numeric 11"(w1983) -> ()
              n1950 = String Length(string=w1984) -> (length=w1986:i32)
              n1951 = Greater?(x=w1986, y=1) -> (0:w1982:bool)
            }
            n1952 = while {
              tunnel: w1964 -> [w1993]
              i -> [w1989]
              stop <- w1988 continue-if-true
              (unwired) TRUE ("line mode (F)")
              n1953 = Read from Text File "Read File"(file (use dialog)=w1993) -> (text=w1990:string)  [unwired: 3 in, 3 out]
              n1954 = local write "Numeric 12"(w1989) -> ()
              n1955 = String Length(string=w1990) -> (length=w1992:i32)
              n1956 = Greater?(x=w1992, y=1) -> (0:w1988:bool)
            }
            n1957 = while {
              tunnel: w1963 -> [w1999]
              i -> [w1995]
              stop <- w1994 continue-if-true
              (unwired) TRUE ("line mode (F)")
              n1958 = Read from Text File "Read File"(file (use dialog)=w1999) -> (text=w1996:string)  [unwired: 3 in, 3 out]
              n1959 = local write "Numeric 13"(w1995) -> ()
              n1960 = String Length(string=w1996) -> (length=w1998:i32)
              n1961 = Greater?(x=w1998, y=1) -> (0:w1994:bool)
            }
            n1962 = String To Path(string=w1962) -> (path=w1970:path)
            n1963 = Open/Create/Replace File "Open File"(file path (use dialog)=w1970) -> (refnum out=w1966:refnum<file>)  [unwired: 5 in, 2 out]
            n1964 = while {
              tunnel: w1966 -> [w1981]
              i -> [w1977]
              stop <- w1976 continue-if-true
              (unwired) TRUE ("line mode (F)")
              n1965 = Read from Text File "Read File"(file (use dialog)=w1981) -> (text=w1978:string)  [unwired: 3 in, 3 out]
              n1966 = local write "Numeric 8"(w1977) -> ()
              n1967 = String Length(string=w1978) -> (length=w1980:i32)
              n1968 = Greater?(x=w1980, y=1) -> (0:w1976:bool)
            }
          }
          frame #1 {
            w2151 = FALSE ("ACTUAL   MERGE")
            # "Sample Temp"
            # "ECR"
            # "COF"
            # "Time\nCOF\nFF\nTemp"
            n1969 = case shown="True" w2024 {
              tunnel: [w2171 w2172] -> w2025
              frame False {
                n1970 = local read "string1"() -> (w2171:string)
              }
              frame True {
                n1971 = local read "String Indicator 4"() -> (w2172:string)
              }
            }
            n1972 = local read "string1 3"() -> (w2069:string)
            n1973 = String To Path(string=w2025) -> (path=w2156:path)
            n1974 = String To Path(string=w2069) -> (path=w2167:path)
            n1975 = local read "Numeric 12"() -> (w2153:i32)
            n1976 = local read "Numeric 8"() -> (w2155:i32)
            n1977 = local read "string1 2"() -> (w2070:string)
            n1978 = local read "string1 4"() -> (w2068:string)
            n1979 = Open/Create/Replace File "Open File"(file path (use dialog)=w2156) -> (refnum out=w2170:refnum<file>, error out=w2169:errorcluster)  [unwired: 5 in, 1 out]
            n1980 = Open/Create/Replace File "Open File"(file path (use dialog)=w2167) -> (refnum out=w2163:refnum<file>, error out=w2164:errorcluster)  [unwired: 5 in, 1 out]
            n1981 = for {
              N: w2155 -> [_]
              tunnel: w2170 -> [w2318]
              tunnel: w2169 -> [w2317]
              tunnel: [w2307] -> w2082 mode=indexing
              tunnel: [w2305] -> w2139 mode=indexing
              tunnel: [w2306] -> w2134 mode=indexing
              tunnel: w2151 -> [_]
              tunnel: [w2299] -> w2136 mode=indexing
              tunnel: [w2295] -> w2105 mode=indexing
              tunnel: [w2291] -> w2080 mode=indexing
              tunnel: [w2287] -> w2061 mode=indexing
              tunnel: [w2282] -> w2021 mode=indexing
              (unwired) TRUE ("line mode (F)")
              # "freq"
              # "Stroke"
              # "Time"
              # "CoF"
              # "Humidity"
              # "Temp"
              # "Air Temp"
              # "ECR"
              n1982 = Read from Text File "Read File"(file (use dialog)=w2318, error in=w2317) -> (text=w2283:string)  [unwired: 2 in, 3 out]
              n1983 = local write "String 6"(w2283) -> ()
              n1984 = String Subset(string=w2283, offset (0)=0, length (rest)=14 ("length (rest)")) -> (substring=w2311:string)
              n1985 = String Subset(string=w2283, offset (0)=35, length (rest)=9 ("length (rest)")) -> (substring=w2308:string)
              n1986 = String Subset(string=w2283, offset (0)=15, length (rest)=9 ("length (rest)")) -> (substring=w2314:string)
              n1987 = Fract/Exp String To Number(string=w2311) -> (number=w2307:dbl)  [unwired: 3 in, 1 out]
              n1988 = Fract/Exp String To Number(string=w2308) -> (number=w2306:dbl)  [unwired: 3 in, 1 out]
              n1989 = Fract/Exp String To Number(string=w2314) -> (number=w2305:dbl)  [unwired: 3 in, 1 out]
              n1990 = String Subset(string=w2283, offset (0)=85, length (rest)=9 ("length (rest)")) -> (substring=w2284:string)
              n1991 = String Subset(string=w2283, offset (0)=25, length (rest)=9 ("length (rest)")) -> (substring=w2290:string)
              n1992 = String Subset(string=w2283, offset (0)=55, length (rest)=9 ("length (rest)")) -> (substring=w2292:string)
              n1993 = String Subset(string=w2283, offset (0)=45, length (rest)=9 ("length (rest)")) -> (substring=w2298:string)
              n1994 = String Subset(string=w2283, offset (0)=65, length (rest)=9 ("length (rest)")) -> (substring=w2304:string)
              n1995 = Fract/Exp String To Number(string=w2290) -> (number=w2287:dbl)  [unwired: 3 in, 1 out]
              n1996 = Fract/Exp String To Number(string=w2284) -> (number=w2282:dbl)  [unwired: 3 in, 1 out]
              n1997 = Fract/Exp String To Number(string=w2292) -> (number=w2291:dbl)  [unwired: 3 in, 1 out]
              n1998 = Fract/Exp String To Number(string=w2298) -> (number=w2295:dbl)  [unwired: 3 in, 1 out]
              n1999 = Fract/Exp String To Number(string=w2304) -> (number=w2301:dbl)  [unwired: 3 in, 1 out]
              n2000 = Add(x=w2301, y=0.0) -> (x+y=w2299:dbl)
            }
            n2001 = for {
              N: w2153 -> [_]
              tunnel: w2164 -> [w2244]
              tunnel: w2163 -> [w2243]
              tunnel: [w2233] -> w2122 mode=indexing
              tunnel: [w2231] -> w2120 mode=indexing
              tunnel: [w2232] -> w2116 mode=indexing
              tunnel: w2151 -> [_]
              tunnel: [w2225] -> w2118 mode=indexing
              tunnel: [w2221] -> w2100 mode=indexing
              tunnel: [w2217] -> w2076 mode=indexing
              tunnel: [w2214] -> w2057 mode=indexing
              tunnel: [w2210] -> w2016 mode=indexing
              (unwired) 9 ("length (rest)")
              (unwired) 9 ("length (rest)")
              (unwired) TRUE ("line mode (F)")
              n2002 = Read from Text File "Read File"(file (use dialog)=w2243, error in=w2244) -> (text=w2211:string)  [unwired: 2 in, 3 out]
              n2003 = local write "String 8"(w2211) -> ()
              n2004 = String Subset(string=w2211, offset (0)=85) -> (substring=w2213:string)  [unwired: 1 in]
              n2005 = String Subset(string=w2211, offset (0)=35, length (rest)=9 ("length (rest)")) -> (substring=w2234:string)
              n2006 = String Subset(string=w2211, offset (0)=55, length (rest)=9 ("length (rest)")) -> (substring=w2219:string)
              n2007 = String Subset(string=w2211, offset (0)=25) -> (substring=w2215:string)  [unwired: 1 in]
              n2008 = String Subset(string=w2211, offset (0)=15, length (rest)=9 ("length (rest)")) -> (substring=w2240:string)
              n2009 = String Subset(string=w2211, offset (0)=0, length (rest)=14 ("length (rest)")) -> (substring=w2237:string)
              n2010 = String Subset(string=w2211, offset (0)=45, length (rest)=9 ("length (rest)")) -> (substring=w2224:string)
              n2011 = String Subset(string=w2211, offset (0)=65, length (rest)=9 ("length (rest)")) -> (substring=w2230:string)
              n2012 = Fract/Exp String To Number(string=w2213) -> (number=w2210:dbl)  [unwired: 3 in, 1 out]
              n2013 = Fract/Exp String To Number(string=w2234) -> (number=w2232:dbl)  [unwired: 3 in, 1 out]
              n2014 = Fract/Exp String To Number(string=w2219) -> (number=w2217:dbl)  [unwired: 3 in, 1 out]
              n2015 = Fract/Exp String To Number(string=w2215) -> (number=w2214:dbl)  [unwired: 3 in, 1 out]
              n2016 = Fract/Exp String To Number(string=w2240) -> (number=w2231:dbl)  [unwired: 3 in, 1 out]
              n2017 = Fract/Exp String To Number(string=w2237) -> (number=w2233:dbl)  [unwired: 3 in, 1 out]
              n2018 = Fract/Exp String To Number(string=w2224) -> (number=w2221:dbl)  [unwired: 3 in, 1 out]
              n2019 = Fract/Exp String To Number(string=w2230) -> (number=w2227:dbl)  [unwired: 3 in, 1 out]
              n2020 = Add(x=w2227, y=0.0) -> (x+y=w2225:dbl)
            }
            n2021 = String To Path(string=w2070) -> (path=w2168:path)
            n2022 = String To Path(string=w2068) -> (path=w2162:path)
            n2023 = local read "Numeric 11"() -> (w2152:i32)
            n2024 = local read "Numeric 13"() -> (w2154:i32)
            n2025 = Open/Create/Replace File "Open File"(file path (use dialog)=w2168) -> (refnum out=w2166:refnum<file>, error out=w2165:errorcluster)  [unwired: 5 in, 1 out]
            n2026 = Open/Create/Replace File "Open File"(file path (use dialog)=w2162) -> (refnum out=w2161:refnum<file>, error out=w2160:errorcluster)  [unwired: 5 in, 1 out]
            n2027 = for {
              N: w2152 -> [_]
              tunnel: w2166 -> [w2281]
              tunnel: w2165 -> [w2280]
              tunnel: [w2270] -> w2132 mode=indexing
              tunnel: [w2268] -> w2130 mode=indexing
              tunnel: [w2269] -> w2125 mode=indexing
              tunnel: w2151 -> [_]
              tunnel: [w2262] -> w2127 mode=indexing
              tunnel: [w2258] -> w2103 mode=indexing
              tunnel: [w2254] -> w2078 mode=indexing
              tunnel: [w2250] -> w2059 mode=indexing
              tunnel: [w2245] -> w2017 mode=indexing
              (unwired) TRUE ("line mode (F)")
              n2028 = Read from Text File "Read File"(file (use dialog)=w2281, error in=w2280) -> (text=w2246:string)  [unwired: 2 in, 3 out]
              n2029 = local write "String 7"(w2246) -> ()
              n2030 = String Subset(string=w2246, offset (0)=85, length (rest)=9 ("length (rest)")) -> (substring=w2249:string)
              n2031 = String Subset(string=w2246, offset (0)=35, length (rest)=9 ("length (rest)")) -> (substring=w2271:string)
              n2032 = String Subset(string=w2246, offset (0)=55, length (rest)=9 ("length (rest)")) -> (substring=w2257:string)
              n2033 = String Subset(string=w2246, offset (0)=25, length (rest)=9 ("length (rest)")) -> (substring=w2251:string)
              n2034 = String Subset(string=w2246, offset (0)=45, length (rest)=9 ("length (rest)")) -> (substring=w2259:string)
              n2035 = String Subset(string=w2246, offset (0)=0, length (rest)=14 ("length (rest)")) -> (substring=w2274:string)
              n2036 = String Subset(string=w2246, offset (0)=15, length (rest)=9 ("length (rest)")) -> (substring=w2277:string)
              n2037 = String Subset(string=w2246, offset (0)=65, length (rest)=9 ("length (rest)")) -> (substring=w2263:string)
              n2038 = Fract/Exp String To Number(string=w2249) -> (number=w2245:dbl)  [unwired: 3 in, 1 out]
              n2039 = Fract/Exp String To Number(string=w2271) -> (number=w2269:dbl)  [unwired: 3 in, 1 out]
              n2040 = Fract/Exp String To Number(string=w2257) -> (number=w2254:dbl)  [unwired: 3 in, 1 out]
              n2041 = Fract/Exp String To Number(string=w2251) -> (number=w2250:dbl)  [unwired: 3 in, 1 out]
              n2042 = Fract/Exp String To Number(string=w2259) -> (number=w2258:dbl)  [unwired: 3 in, 1 out]
              n2043 = Fract/Exp String To Number(string=w2274) -> (number=w2270:dbl)  [unwired: 3 in, 1 out]
              n2044 = Fract/Exp String To Number(string=w2277) -> (number=w2268:dbl)  [unwired: 3 in, 1 out]
              n2045 = Fract/Exp String To Number(string=w2263) -> (number=w2266:dbl)  [unwired: 3 in, 1 out]
